vi "Msg.vi"(7 "Actor in":refnum<class "Actor.lvclass">, 11 "Override Error Msg in":refnum<class "Override Error Msg.lvclass">) -> (5 "Actor out":refnum<class "Actor.lvclass">)   [LabVIEW 2021, in "Override Error.lvlib" / "Override Error Msg.lvclass"]
uses:
  Override Error Msg.lvclass
  Override Error/Override Error.lvclass
  Merge Error/Merge Error/Merge Error.lvclass
  Actor/Actor.lvclass
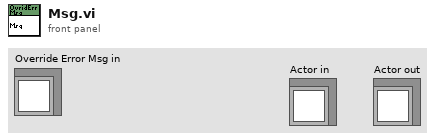
[diagram p1: front panel]
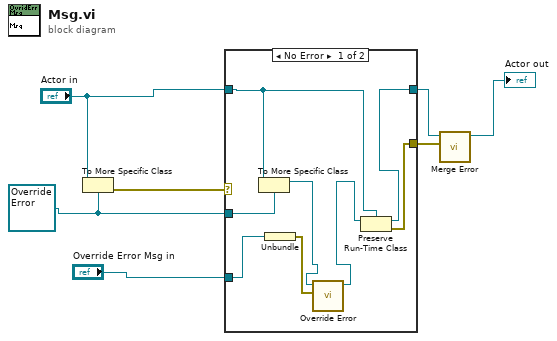
[diagram p0: block diagram]
diagram:
  w3 = refnum<class "Override Error.lvclass"> refnum ("Override Error.lvlib:Override Error.lvclass")
  n1 = To More Specific Class(target class=w3, reference="Actor in") -> (error out=w7:errorcluster)  [unwired: 1 in, 1 out]
  n2 = case shown="No Error" w7 {
    selector: w7 -> [_ w16]
    tunnel: [w9 w17] -> w6
    tunnel: "Actor in" -> [w11 w17]
    tunnel: w3 -> [w15 _]
    tunnel: "Override Error Msg in" -> [w13 _]
    tunnel: [w8 w16] -> w5
    frame No Error {
      n3 = To More Specific Class(target class=w15, reference=w11) -> (specific class reference=w14:refnum<class "Override Error.lvclass">)  [unwired: 1 in, 1 out]
      n4 = Unbundle(w13) -> (w12:errorcluster)
      n5 = call-dynamic "Override Error.vi"("Error"=w12, "Override Error in"=w14) -> ("Override Error out"=w10:refnum<class "Override Error.lvclass">)  [unwired: 9 in]
      n6 = Preserve Run-Time Class(object in=w10, 2:w11) -> (object out=w9:refnum<class "Actor.lvclass">, error out=w8:errorcluster)  [unwired: 1 in]
    }
    frame Error {
    }
  }
  n7 = call-dynamic "Merge Error.vi"("Error"=w5, "Set Error in"=w6) -> ("Set Error out"=→"Actor out":refnum<class "Merge Error.lvclass">)  [unwired: 9 in]
